vi "GetParam.vi"(8 "error in (no error)":errorcluster caption="entrée d'erreur (pas d'erreur)", 11 "Silhouette_Samples.lvclass":refnum<class "Silhouette_Samples.lvclass">) -> (0 "error out":errorcluster caption="sortie d'erreur", 2 "silhouette_samples":cluster{"metric":string}={"metric"="euclidean"}, 3 "Silhouette_Samples.lvclass":refnum<class "Silhouette_Samples.lvclass">)   [LabVIEW 2020, in "Silhouette_Samples.lvclass"]
doc: "Get Parameters"
uses:
  Silhouette_Samples.lvclass
  Silhouette_Samples.lvclass/Silhouette_Samples.ctl
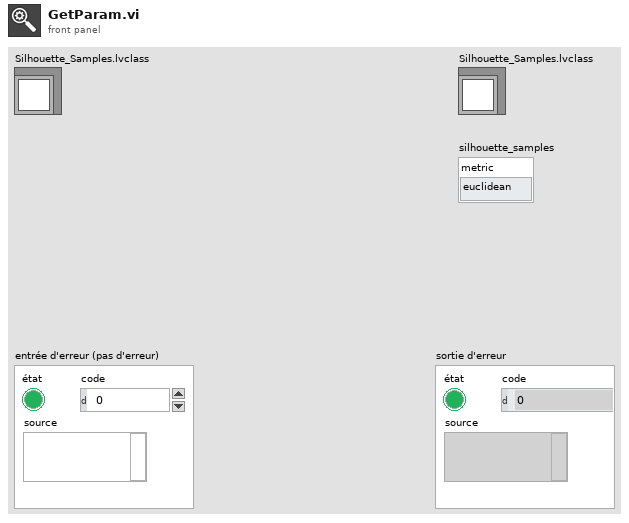
[diagram p1: front panel]
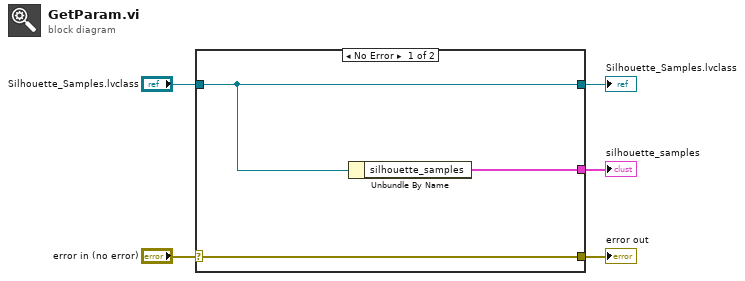
[diagram p0: block diagram]
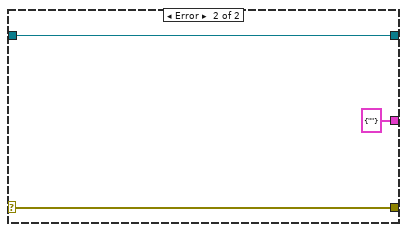
[diagram p2: hidden frame]
diagram:
  n1 = case shown="No Error" "error in (no error)" {
    selector: "error in (no error)" -> [w8 w10]
    tunnel: [w8 w10] -> w4
    tunnel: [w7 w11] -> w2
    tunnel: "Silhouette_Samples.lvclass" -> [w7 w11]
    tunnel: [w6 cluster{"metric":string} {"metric"=""} ("silhouette_samples")] -> w1
    frame No Error {
      n2 = Unbundle By Name(w7) -> ("silhouette_samples"=w6:cluster{"metric":string})
    }
    frame Error {
    }
  }
  "error out" <- w4
  "Silhouette_Samples.lvclass" <- w2
  "silhouette_samples" <- w1
